vi "Handle Command.vi"(8 "error in (no error)":errorcluster, 9 "params in":variant, 10 "command":string, 11 "Inst.Transport in":refnum<class "Inst.Transport.lvclass">) -> (0 "error out":errorcluster, 1 "processed data":variant, 2 "command out":string, 3 "Inst.Transport out":refnum<class "Inst.Transport.lvclass">)   [LabVIEW 2019, in "Inst.Transport.lvclass"]
uses:
  Inst.Transport.lvclass
  Inst.Transport.lvclass/Inst.Transport.ctl
  Typedefs/getStatus--Reply--Cluster.ctl
  Typedefs/Inst.Transport.Status--Enum.ctl
  <userlib>/LevyLab/Instrument Framework/Instrument Types/SCPI/Instrument.SCPI.lvclass
  Typedefs/Inst.Transport.PublicCommands--Enum.ctl
  Typedefs/Inst.Transport.ProtectedCommands--Enum.ctl
  552737b8-b1ca-46ed-8e29-167e2822ff5d.vi
  25d97d38-0eab-472e-b12a-584ad5c8b013.vi
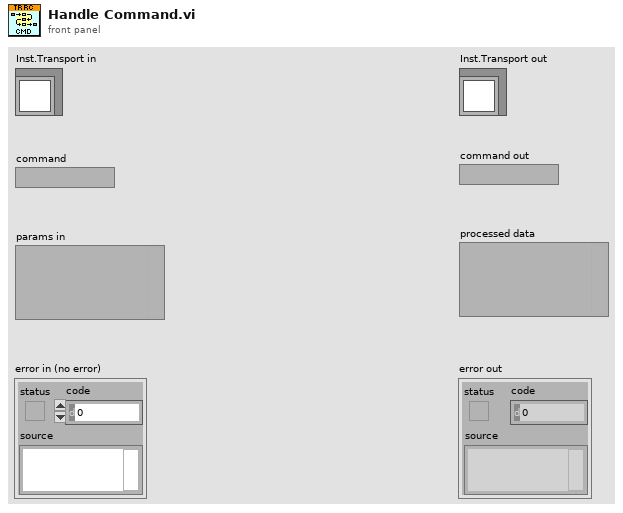
[diagram p1: front panel]
types:
  T1 = typedef "Inst.Transport.lvclass/getStatus--Reply--Cluster.ctl" = cluster{"Status":T2}
  T2 = typedef "Inst.Transport.lvclass/Inst.Transport.Status--Enum.ctl" = enum16{"idle", "running"}
  T3 = typedef "Inst.Transport.lvclass/Inst.Transport.PublicCommands--Enum.ctl" = enum16{"startTransport", "stopTransport", "getStatus", "setExptFolder", "setExptComments", "appendExptParam", "clearExptParam", "setExptParam", "setSweepConfig"}
  T4 = typedef "Inst.Transport.lvclass/Inst.Transport.ProtectedCommands--Enum.ctl" = enum16{"setStatus", "showUI", "hideUI"}
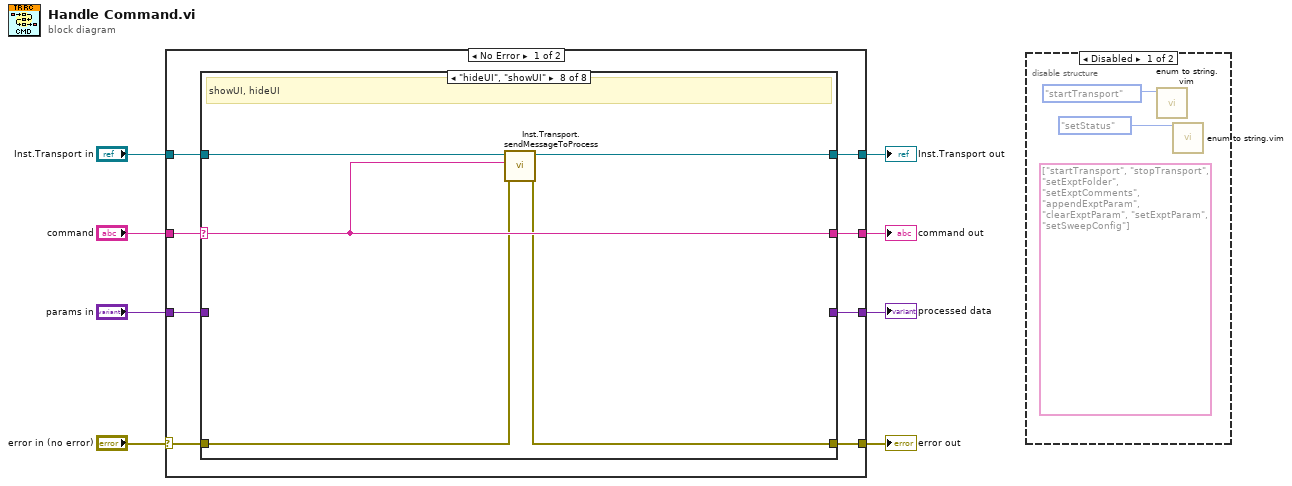
[diagram p0: block diagram]
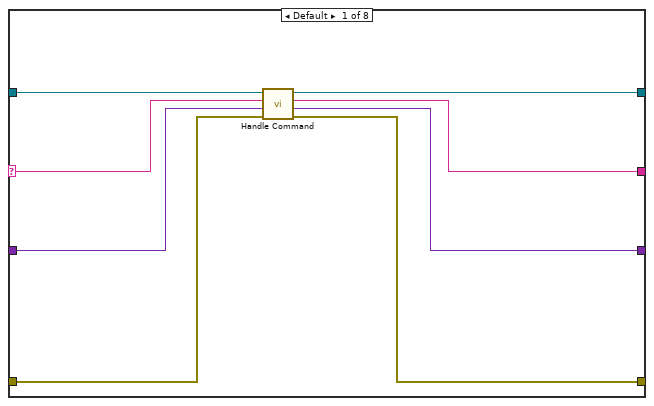
[diagram p3: hidden frame]
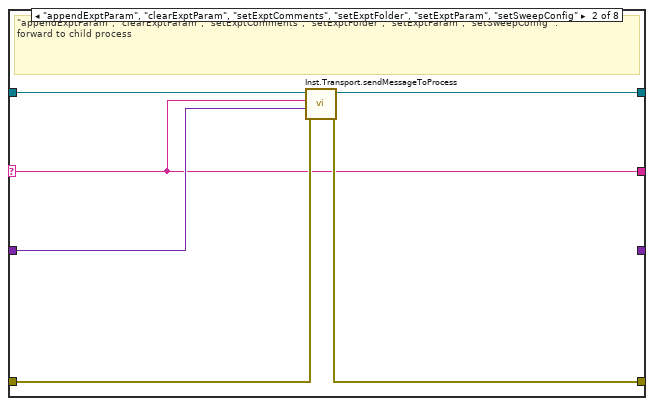
[diagram p4: hidden frame]
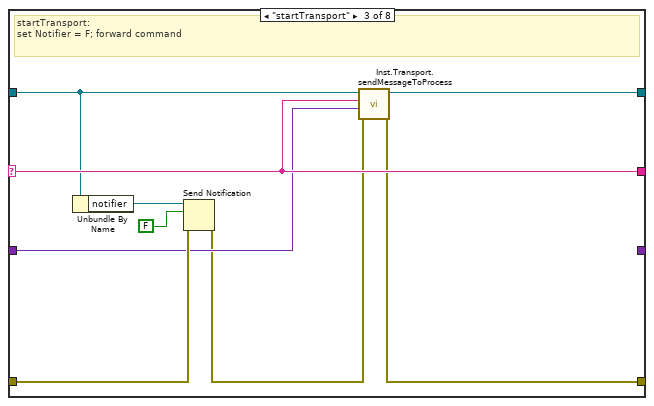
[diagram p5: hidden frame]
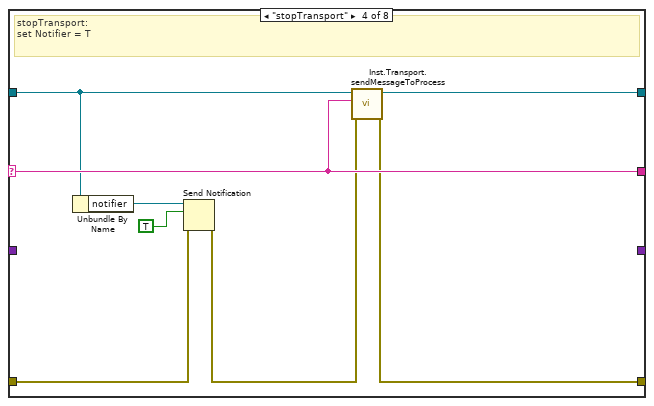
[diagram p6: hidden frame]
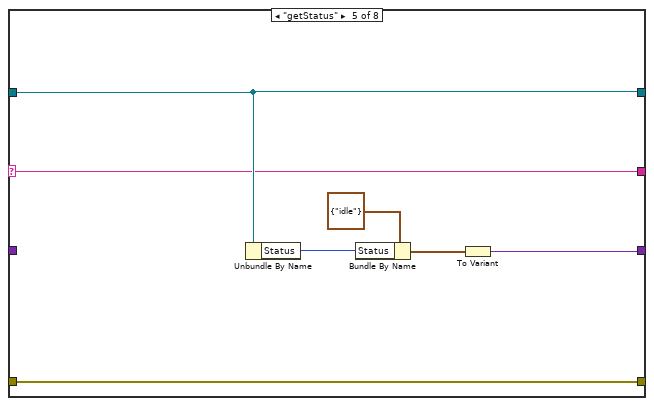
[diagram p7: hidden frame]
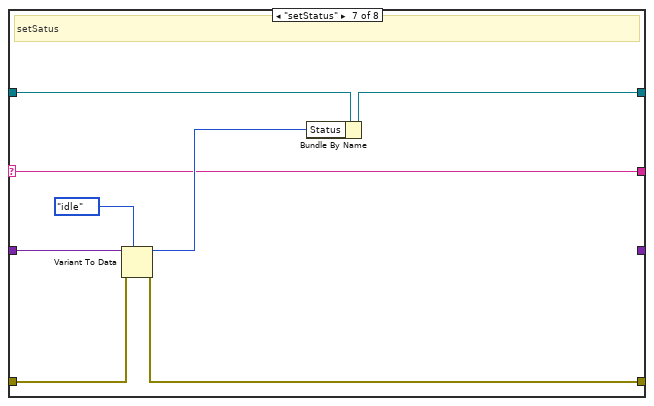
[diagram p9: hidden frame]
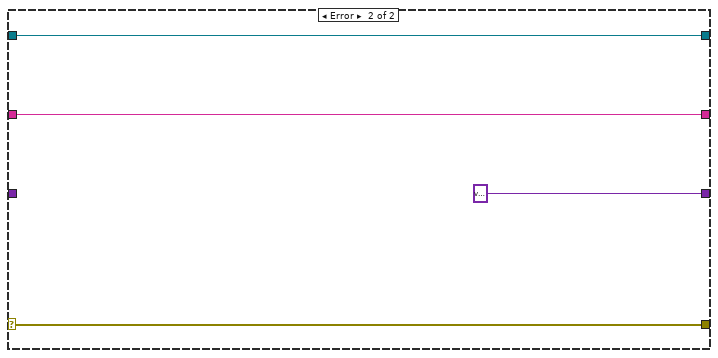
[diagram p10: hidden frame]
diagram:
  n1 = case shown="No Error" "error in (no error)" {
    selector: "error in (no error)" -> [w11 w73]
    tunnel: [w9 w73] -> w6
    tunnel: [w14 w72] -> w5
    tunnel: "Inst.Transport in" -> [w15 w72]
    tunnel: "command" -> [w16 w71]
    tunnel: [w13 variant ("Variant")] -> w3
    tunnel: "params in" -> [w10 _]
    tunnel: [w12 w71] -> w1
    frame No Error {
      n2 = case shown="\"hideUI\", \"showUI\"" w16 {
        selector: w16 -> [w18 w25 w36 w43 w48 _ w57 w67]
        tunnel: w15 -> [w22 w30 w31 w42 w54 w56 w64 w69]
        tunnel: [w19 w29 w32 w44 w54 w56 w63 w68] -> w14
        tunnel: [w21 _ _ _ w53 _ _ _] -> w13
        tunnel: w11 -> [w23 w28 w37 w45 w52 w55 w59 w66]
        tunnel: w10 -> [w24 w26 w35 _ _ _ w61 _]
        tunnel: [w17 w25 w36 w43 w48 _ w57 w67] -> w12
        tunnel: [w20 w27 w33 w40 w52 w55 w58 w65] -> w9
        frame Default {
          n3 = call-parent "Handle Command.vi"("error in (no error)"=w23, "params in"=w24, "command"=w18, "Instrument in"=w22) -> ("error out"=w20:errorcluster, "processed data"=w21:variant, "command out"=w17:string, "Instrument out"=w19:refnum<class "Inst.Transport.lvclass">)  [unwired: 4 in]
        }
        frame "appendExptParam", "clearExptParam", "setExptComments", "setExptFolder", "setExptParam", "setSweepConfig" {
          # "\"appendExptParam\", \"clearExptParam\", \"setExptComments\", \"setExptFolder\", \"setExptParam\", \"setSweepConfig\" :\nforward to child process"
          n4 = call "Inst.Transport.sendMessageToProcess.vi"("error in (no error)"=w28, "Data"=w26, "Command"=w25, "Inst.Transport in"=w30) -> ("error out"=w27:errorcluster, "Inst.Transport out"=w29:refnum<class "Inst.Transport.lvclass">)  [unwired: 6 in]
        }
        frame "startTransport" {
          # "startTransport:\nset Notifier = F; forward command"
          n5 = Unbundle By Name(w31) -> ("notifier"=w39:refnum<notifier>)
          n6 = Send Notification(notification=FALSE, notifier=w39, error in (no error)=w37) -> (error out=w34:errorcluster)  [unwired: 1 out]
          n7 = call "Inst.Transport.sendMessageToProcess.vi"("error in (no error)"=w34, "Data"=w35, "Command"=w36, "Inst.Transport in"=w31) -> ("error out"=w33:errorcluster, "Inst.Transport out"=w32:refnum<class "Inst.Transport.lvclass">)  [unwired: 6 in]
        }
        frame "stopTransport" {
          # "stopTransport:\nset Notifier = T"
          n8 = Unbundle By Name(w42) -> ("notifier"=w47:refnum<notifier>)
          n9 = Send Notification(notification=TRUE, notifier=w47, error in (no error)=w45) -> (error out=w41:errorcluster)  [unwired: 1 out]
          n10 = call "Inst.Transport.sendMessageToProcess.vi"("error in (no error)"=w41, "Command"=w43, "Inst.Transport in"=w42) -> ("error out"=w40:errorcluster, "Inst.Transport out"=w44:refnum<class "Inst.Transport.lvclass">)  [unwired: 7 in]
        }
        frame "getStatus" {
          n11 = Unbundle By Name(w54) -> ("Status"=w50:T2)
          n12 = Bundle By Name(cluster=T1 {"Status"=enum."idle"} ("getStatus"), "Status"=w50) -> (w49:T1)
          n13 = To Variant(anything=w49) -> (Variant=w53:variant)
        }
        frame "---Protected Methods---" {
        }
        frame "setStatus" {
          # "setSatus"
          n14 = Variant To Data(error in=w59, type=Inst.Transport.Status--Enum."idle" ("Status"), Variant=w61) -> (data=w62:T2, error out=w58:errorcluster)
          n15 = Bundle By Name(cluster=w64, "Status"=w62) -> (w63:refnum<class "Inst.Transport.lvclass">)
        }
        frame "hideUI", "showUI" {
          # "showUI, hideUI"
          n16 = call "Inst.Transport.sendMessageToProcess.vi"("error in (no error)"=w66, "Command"=w67, "Inst.Transport in"=w69) -> ("error out"=w65:errorcluster, "Inst.Transport out"=w68:refnum<class "Inst.Transport.lvclass">)  [unwired: 7 in]
        }
      }
    }
    frame Error {
    }
  }
  "error out" <- w6
  "Inst.Transport out" <- w5
  "command out" <- w1
  "processed data" <- w3
  n17 = disable-structure shown="Disabled" {
    frame Disabled {
      (unwired) string[] ["startTransport", "stopTransport", "setExptFolder", "setExptComments", "appendExptParam", "clearExptParam", "setExptParam", "setSweepConfig"] ("Commands")
      n18 = call "enum to string.vim"("enum in"=Inst.Transport.PublicCommands--Enum."startTransport" ("PublicCommands")) -> ()  [unwired: 9 in, 2 out]
      n19 = call "enum to string.vim"("enum in"=Inst.Transport.ProtectedCommands--Enum."setStatus" ("ProtectedCommands")) -> ()  [unwired: 9 in, 2 out]
    }
    frame Enabled {
    }
  }
